vi "Tosca-Initialize SCL.vi"(0 "Schedule":T4, 5 "Block":i32, 7 "previous order":i32[](array[numeric]), 9 "Mode":T1) -> (4 "SCL":T2[](array[typedef]), 8 "order":i32[](array[numeric]))   [LabVIEW 2020]
uses:
  Typedefs/Tosca-Schedule.ctl
  Typedefs/Tosca-Sequence Order.ctl
  Typedefs/Tosca-Parameter Family.ctl
  Typedefs/Tosca-Parameter Table Element.ctl
  Typedefs/Tosca-Parameter Dimension.ctl
  Typedefs/Tosca-SCL Element.ctl
  Typedefs/Tosca-Schedule Mode.ctl
  Typedefs/Tosca-Event Type.ctl
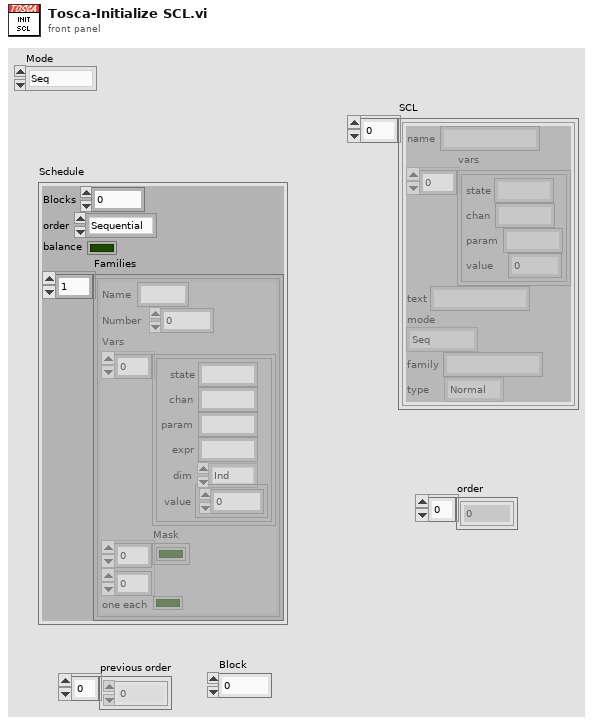
[diagram p1: front panel]
types:
  T1 = typedef "Tosca-Schedule Mode.ctl" = enum16{"Seq", "CS+/CS-", "Adapt"}
  T2 = typedef "Tosca-SCL Element.ctl" = cluster{"name":string, "vars":cluster{"state":string, "chan":string, "param":string, "value":dbl}[], "text":string, "mode":T1, "family":string, "type":T3}
  T3 = typedef "Tosca-Event Type.ctl" = enum16{"Normal", "CS+", "CS-"}
  T4 = typedef "Tosca-Schedule.ctl" = cluster{"Blocks":i32, "order":T5, "balance":bool, "Families":T6[]}
  T5 = typedef "Tosca-Sequence Order.ctl" = enum16{"Sequential", "Alternate", "Randomize", "Random group"}
  T6 = typedef "Tosca-Parameter Family.ctl" = cluster{"Name":string, "Number":i32, "Vars":T7[], "Mask":bool[][], "one each":bool}
  T7 = typedef "Tosca-Parameter Table Element.ctl" = cluster{"state":string, "chan":string, "param":string, "expr":string, "dim":T8, "value":dbl[]}
  T8 = typedef "Tosca-Parameter Dimension.ctl" = enum16{"Ind", "X", "Y"}
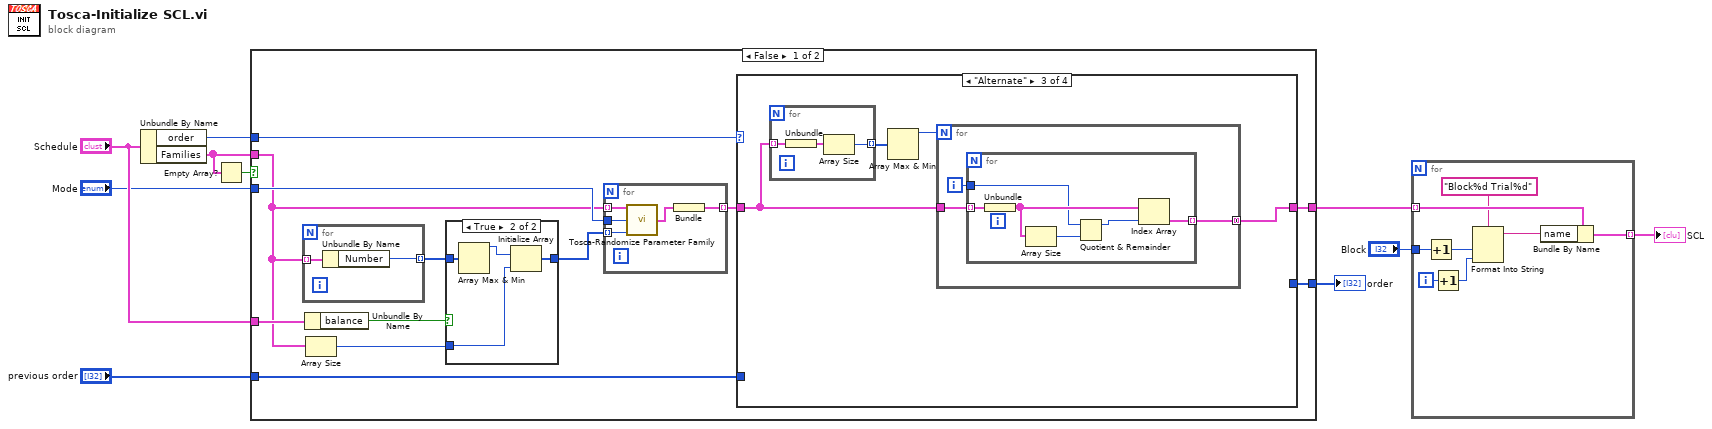
[diagram p0: block diagram]
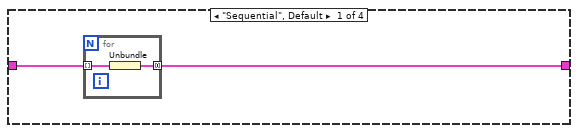
[diagram p3: hidden frame]
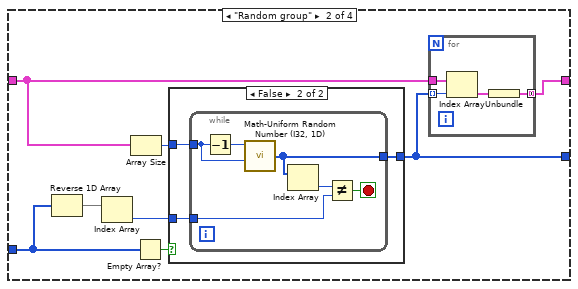
[diagram p4: hidden frame]
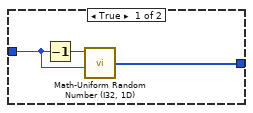
[diagram p5: hidden frame]
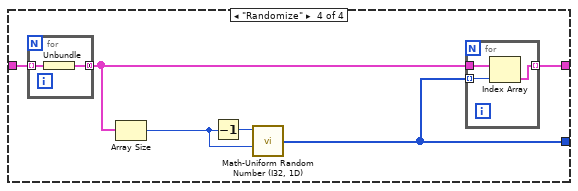
[diagram p6: hidden frame]
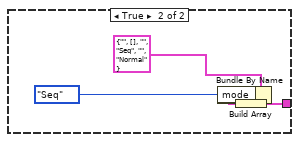
[diagram p7: hidden frame]
diagram:
  n1 = Unbundle By Name("Schedule") -> ("order"=w10:T5, "Families"=w8:T6[])
  n2 = Empty Array?(array=w8) -> (empty?=w5:bool)
  n3 = case shown="False" w5 {
    tunnel: "Schedule" -> [w22 _]
    tunnel: w10 -> [w11 _]
    tunnel: "Mode" -> [w21 _]
    tunnel: w8 -> [w12 _]
    tunnel: [w15 w91] -> w7
    tunnel: [w14 _] -> w3
    tunnel: "previous order" -> [w13 _]
    frame False {
      n4 = for {
        tunnel: w12 -> [w34] mode=indexing
        tunnel: [w33] -> w20 mode=indexing
        n5 = Unbundle By Name(w34) -> ("Number"=w33:i32)
      }
      n6 = Unbundle By Name(w22) -> ("balance"=w19:bool)
      n7 = Array Size(array=w12) -> (size(s)=w17:i32)
      n8 = case shown="True" w19 {
        tunnel: w20 -> [w23 w27]
        tunnel: [w23 w25] -> w18
        tunnel: w17 -> [_ w24]
        frame False {
        }
        frame True {
          n9 = Array Max & Min(array=w27) -> (max value=w26:i32)  [unwired: 3 out]
          n10 = Initialize Array(w26, w24) -> (w25:i32[])
        }
      }
      n11 = for {
        tunnel: w12 -> [w32] mode=indexing
        tunnel: w18 -> [w31] mode=indexing
        tunnel: [w29] -> w16 mode=indexing
        tunnel: w21 -> [w30]
        n12 = call "Tosca-Randomize Parameter Family.vi"("Family in"=w32, "Mode"=w30, "N"=w31) -> ("SCL"=w28:T2[])  [unwired: 11 in, 1 out]
        n13 = Bundle("SCL"=w28) -> (w29:cluster{"SCL":T2[]})  [unwired: 1 in]
      }
      n14 = case shown="\"Alternate\"" w11 {
        tunnel: w16 -> [w36 w40 w65 w82]
        tunnel: [w35 w39 w63 w83] -> w15
        tunnel: [_ w41 _ w80] -> w14
        tunnel: w13 -> [_ w45 _ _]
        frame "Sequential", Default {
          n15 = for {
            tunnel: w36 -> [w37] mode=indexing
            tunnel: [w38] -> w35 mode=concatenating
            n16 = Unbundle(w37) -> ("SCL"=w38:T2[])
          }
        }
        frame "Random group" {
          n17 = Reverse 1D Array(array=w45) -> (reversed array=w46:i32[])
          n18 = Index Array(array=w46) -> (element=w43:i32)  [unwired: 1 in]
          n19 = Array Size(array=w40) -> (size(s)=w42:i32)
          n20 = Empty Array?(array=w45) -> (empty?=w44:bool)
          n21 = case shown="False" w44 {
            tunnel: w42 -> [w52 w56]
            tunnel: [w51 w55] -> w41
            tunnel: w43 -> [_ w54]
            frame True {
              n22 = Decrement(x=w52) -> (x-1=w53:i32)
              n23 = call "Math-Uniform Random Number (I32, 1D).vi"("N"=w52, "Ymax"=w53) -> ("Random Ints"=w51:i32[])  [unwired: 4 in]
            }
            frame False {
              n24 = while {
                tunnel: w56 -> [w61]
                tunnel: [w60] -> w55
                tunnel: w54 -> [w58]
                stop <- w57 stop-if-true
                n25 = Decrement(x=w61) -> (x-1=w62:i32)
                n26 = call "Math-Uniform Random Number (I32, 1D).vi"("N"=w61, "Ymax"=w62) -> ("Random Ints"=w60:i32[])  [unwired: 4 in]
                n27 = Index Array(array=w60) -> (element=w59:i32)  [unwired: 1 in]
                n28 = Not Equal?(x=w59, y=w58) -> (x != y?=w57:bool)
              }
            }
          }
          n29 = for {
            tunnel: w41 -> [w50] mode=indexing
            tunnel: w40 -> [w49]
            tunnel: [w47] -> w39 mode=concatenating
            n30 = Index Array(array=w49, index=w50) -> (element=w48:cluster{"SCL":T2[]})
            n31 = Unbundle(w48) -> ("SCL"=w47:T2[])
          }
        }
        frame "Alternate" {
          n32 = for {
            tunnel: w65 -> [w78] mode=indexing
            tunnel: [w76] -> w66 mode=indexing
            n33 = Unbundle(w78) -> ("SCL"=w77:T2[])
            n34 = Array Size(array=w77) -> (size(s)=w76:i32)
          }
          n35 = Array Max & Min(array=w66) -> (max value=w64:i32)  [unwired: 3 out]
          n36 = for {
            N: w64 -> [_]
            tunnel: w65 -> [w69]
            tunnel: [w68] -> w63 mode=concatenating
            i -> [w67]
            n37 = for {
              tunnel: w69 -> [w75] mode=indexing
              tunnel: [w71] -> w68 mode=indexing
              tunnel: w67 -> [w70]
              n38 = Unbundle(w75) -> ("SCL"=w73:T2[])
              n39 = Array Size(array=w73) -> (size(s)=w74:i32)
              n40 = Quotient & Remainder(x=w70, y=w74) -> (x-y*floor(x/y)=w72:i32)  [unwired: 1 out]
              n41 = Index Array(array=w73, index=w72) -> (element=w71:T2)
            }
          }
        }
        frame "Randomize" {
          n42 = for {
            tunnel: w82 -> [w86] mode=indexing
            tunnel: [w85] -> w81 mode=concatenating
            n43 = Unbundle(w86) -> ("SCL"=w85:T2[])
          }
          n44 = Array Size(array=w81) -> (size(s)=w84:i32)
          n45 = Decrement(x=w84) -> (x-1=w79:i32)
          n46 = call "Math-Uniform Random Number (I32, 1D).vi"("N"=w84, "Ymax"=w79) -> ("Random Ints"=w80:i32[])  [unwired: 4 in]
          n47 = for {
            tunnel: w81 -> [w89]
            tunnel: [w88] -> w83 mode=indexing
            tunnel: w80 -> [w87] mode=indexing
            n48 = Index Array(array=w89, index=w87) -> (element=w88:T2)
          }
        }
      }
    }
    frame True {
      n49 = Bundle By Name(cluster=T2 {"name"="", "vars"=[], "text"="", "mode"=enum."Seq", "family"="", "type"=enum."Normal"} ("StimCon"), "mode"=Tosca-Schedule_Mode."Seq") -> (w92:T2)
      n50 = Build Array(w92) -> (w91:T2[])
    }
  }
  "order" <- w3
  n51 = for {
    tunnel: w7 -> [w101] mode=indexing
    tunnel: [w100] -> w9 mode=indexing
    tunnel: "Block" -> [w98]
    i -> [w97]
    n52 = Increment(x=w98) -> (x+1=w94:i32)
    n53 = Increment(x=w97) -> (x+1=w95:i32)
    n54 = Format Into String(format string="Block%d Trial%d", w94, w95) -> (resulting string=w99:string)  [unwired: 2 in, 1 out]
    n55 = Bundle By Name(cluster=w101, "name"=w99) -> (w100:T2)
  }
  "SCL" <- w9
